vi "DA Output Source.vi"(8 "error in (no error)":errorcluster, 10 "j (0)":T1, 11 "VISA resource name":refnum<visa-resource-name>) -> (0 "error out":errorcluster, 3 "VISA resource name out":refnum<visa-resource-name>)   [LabVIEW 2015, in "SR400.lvlib"]
doc: "AS { j }\nThe AS command reads and sets the front panel\nD/A output source. If j is absent, the D/A source is\nreturned. The parameter j may only be included if\nthe counting mode is A,B FOR T PRESET. In this\ncase, j=0 or 1 selects A or B. In all other modes,\nthe D/A output follows the count display. The\nsource may be read in all modes.\nj Output source\n0 A\n1 B\n2 A-B\n3 A+B"
uses:
  SR400.lvlib
  Typedefs/Output Source.ctl
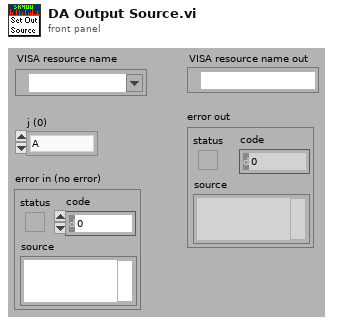
[diagram p1: front panel]
types:
  T1 = typedef "SR400.lvlib/Output Source.ctl" = enum16{"A", "B", "A - B", "A + B"}
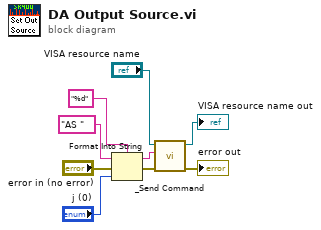
[diagram p0: block diagram]
diagram:
  n1 = Format Into String(format string="%d", initial string="AS " ("command"), error in="error in (no error)", "j (0)") -> (resulting string=w4:string, error out=w3:errorcluster)
  n2 = call "_Send Command.vi"("error in (no error)"=w3, "Command"=w4, "VISA resource name"="VISA resource name") -> ("error out"=→"error out":errorcluster, "VISA resource name out"=→"VISA resource name out":refnum<visa-resource-name>)  [unwired: 1 in, 6 out]
